vi "Main.vi"(11 "Module Admin":refnum<class "Delacor_lib_QMH_Cloneable Module Admin.lvclass">) -> ()   [LabVIEW 2024, in "Thermal Chamber.lvlib"]
doc: "This template is based off of the Queued Message Handler design pattern and the Queued Message Handler project template that ships with LabVIEW.\n\nThe main difference is that the queue is private to this module and communication between modules is performed via Broadcast and Request events.\n\nRequest events are wrapped in public API methods and are handled in the Event Handling Loop (EHL) of this VI. Any module can register for Broadcast events sent by this module. The EHL generates messages based on user interface actions.\n\nThe Message Handling Loop (MHL) processes messages generated by the EHL, or by other messages. The messages are string values, so new messages can be added easily to the Message Cases case structure in the MHL. Each message cluster can also provide an optional value for Message Data, which is a variant that can be converted to whatever message-specific data is required.\n_____\nBased on DQMH Project Template 6.0.0.91.\n\n<b>Note:</b> This VI was modified by the <b>Validate DQMH Module</b> tool to add a 'Panel Hidden' status updated broadcast to the Panel Close? event when External Launch = TRUE.\n\n<b>Note:</b> This VI was modified by the <b>Validate DQMH Module</b> tool to add a call to the Error Reported VI at the end of the 'Exit' MHL frame."
uses:
  Thermal Chamber.lvlib
  <vilib>/Delacor/Delacor QMH/Libraries/Cloneable Module Admin_class/Delacor_lib_QMH_Cloneable Module Admin.lvclass
  C:/Program Files/National Instruments/LabVIEW 2024/vi.lib/Delacor/Delacor QMH/Libraries/Module Admin_class/Delacor_lib_QMH_Module Admin.lvclass
  Module Data--cluster.ctl
  Class Libraries/Process Controller/_Thermal Process Controller.lvclass
  <vilib>/Delacor/Delacor QMH/Libraries/Message Queue_class/Delacor_lib_QMH_Message Queue.lvclass/Delacor_lib_QMH_Message Queue.ctl
  <vilib>/Delacor/Delacor QMH/Libraries/Cloneable Module Admin_class/Delacor_lib_QMH_Cloneable Module Admin.lvclass/Delacor_lib_QMH_Cloneable Module Admin.ctl
  Stop Argument--cluster.ctl
  <vilib>/Delacor/Delacor QMH/Libraries/Module Admin_class/Delacor_lib_QMH_Module Admin.lvclass/Delacor_lib_QMH_Module Admin.ctl
  Initialize Argument--cluster.ctl
  Class Libraries/Process Controller/Controls/Class Selector--Enum.ctl
  Initialize (Reply Payload)--cluster.ctl
  Shutdown Argument--cluster.ctl
  Shutdown (Reply Payload)--cluster.ctl
  Set Temp Setpoint Argument--cluster.ctl
  Class Libraries/Process Controller/Controls/Temp Data--Cluster.ctl
  Class Libraries/Process Controller/Controls/Temperature Units--Enum.ctl
  Set Temp Setpoint (Reply Payload)--cluster.ctl
  Set Temp Ramp Rate Argument--cluster.ctl
  Class Libraries/Process Controller/Controls/Temp Ramp Rate Data--Cluster.ctl
  Class Libraries/Process Controller/Controls/Rate Units--Enum.ctl
  Set Temp Ramp Rate (Reply Payload)--cluster.ctl
  Set Temp Control State Argument--cluster.ctl
  Set Temp Control State (Reply Payload)--cluster.ctl
  Get Temp Feedback Argument--cluster.ctl
  Get Temp Feedback (Reply Payload)--cluster.ctl
  Read Controller Data Argument--cluster.ctl
  Read Controller Data (Reply Payload)--cluster.ctl
  <vilib>/Utility/miscctls.llb/LVPointTypeDef.ctl
  Class Libraries/Simulated Process Controller/Simulated Thermal Process Controller.lvclass
  C:/Users/ghahn/OneDrive - Milwaukee Tool/Documents/LabVIEW Data/CML DQMH/Libraries/Thermal Chamber/Class Libraries/Process Controller/_Thermal Process Controller.lvclass
  Class Libraries/Watlow F4T/Watlow F4T.lvclass
  <vilib>/Delacor/Delacor QMH/Libraries/Message Queue_class/Delacor_lib_QMH_Enqueue Message (Single).vi
  <vilib>/Delacor/Delacor QMH/Libraries/Cloneable Module Admin_class/Delacor_lib_QMH_Get Module ID.vi
  <vilib>/Delacor/Delacor QMH/Libraries/Module Admin_class/Delacor_lib_QMH_Get External Launch.vi
  <vilib>/Utility/error.llb/Error Cluster From Error Code.vi
  <vilib>/ErrorRing/Error Ring.xnode
  <vilib>/Delacor/Delacor QMH/Libraries/Message Queue_class/Delacor_lib_QMH_Message Queue.lvclass
panel:
  out "Module ID":i32=-1
  out "error out":errorcluster
  out "Status":string
  in  "Simulate EHL Error":bool
  in  "Simulate MHL Error":bool
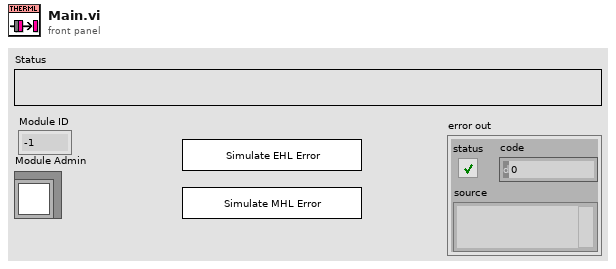
[diagram p1: front panel]
types:
  T1 = typedef "Thermal Chamber.lvlib/Request Events--cluster.ctl" = cluster{"Stop Module":refnum<user-event>, "Show Panel":refnum<user-event>, "Hide Panel":refnum<user-event>, "Show Diagram":refnum<user-event>, "Get Module Execution Status":refnum<user-event>, "Initialize":refnum<user-event>, "Shutdown":refnum<user-event>, "Set Temp Setpoint":refnum<user-event>, "Set Temp Ramp Rate":refnum<user-event>, "Set Temp Control State":refnum<user-event>, "Get Temp Feedback":refnum<user-event>, "Read Controller Data":refnum<user-event>}
  T2 = typedef "Thermal Chamber.lvlib/Module Data--cluster.ctl" = cluster{"Status":string, "_Thermal Process Controller":refnum<class "_Thermal Process Controller.lvclass">}
  T3 = enum32{"invalid lock state", "Not Locked", "Locked (No Password)", "Password-protected"}
  T4 = typedef "Thermal Chamber.lvlib/Stop Argument--cluster.ctl" = cluster{"Module ID":i32, "Origin":string, "Exit via Stop Module Req?":bool, "Wait for Module to stop?":bool}
  T5 = typedef "Thermal Chamber.lvlib/Initialize Argument--cluster.ctl" = cluster{"Module ID":i32, "Class Types":T6, "VISA":refnum<visa-resource-name>, "Wait Notifier":refnum<notifier>, "wait for reply":bool}
  T6 = typedef "_Thermal Process Controller.lvclass/Class Selector--Enum.ctl" = enum16{"Simulated Thermal Process Controller", "Watlow F4T"}
  T7 = typedef "Thermal Chamber.lvlib/Shutdown Argument--cluster.ctl" = cluster{"Module ID":i32, "Wait Notifier":refnum<notifier>, "wait for reply":bool}
  T8 = typedef "Thermal Chamber.lvlib/Set Temp Setpoint Argument--cluster.ctl" = cluster{"Module ID":i32, "Temp Setpoint Data":T9, "Wait Notifier":refnum<notifier>, "wait for reply":bool}
  T9 = typedef "_Thermal Process Controller.lvclass/Temp Data--Cluster.ctl" = cluster{"Temp":dbl, "Temp Units":T10}
  T10 = typedef "_Thermal Process Controller.lvclass/Temperature Units--Enum.ctl" = enum16{"Degrees F", "Degrees C", "Degrees K"}
  T11 = typedef "Thermal Chamber.lvlib/Set Temp Ramp Rate Argument--cluster.ctl" = cluster{"Module ID":i32, "Temp Ramp Data":T12, "Wait Notifier":refnum<notifier>, "wait for reply":bool}
  T12 = typedef "_Thermal Process Controller.lvclass/Temp Ramp Rate Data--Cluster.ctl" = cluster{"Temp Ramp Rate":dbl, "Temp Units":T10, "Rate Units":T13}
  T13 = typedef "_Thermal Process Controller.lvclass/Rate Units--Enum.ctl" = enum16{"Degrees/Minutes", "Degrees/Hours"}
  T14 = typedef "Thermal Chamber.lvlib/Set Temp Control State Argument--cluster.ctl" = cluster{"Module ID":i32, "State":bool, "Wait Notifier":refnum<notifier>, "wait for reply":bool}
  T15 = typedef "Thermal Chamber.lvlib/Get Temp Feedback Argument--cluster.ctl" = cluster{"Module ID":i32, "Temp Units":T10, "Wait Notifier":refnum<notifier>, "wait for reply":bool}
  T16 = typedef "Thermal Chamber.lvlib/Read Controller Data Argument--cluster.ctl" = cluster{"Module ID":i32, "Temp Units":T10, "Wait Notifier":refnum<notifier>, "wait for reply":bool}
  T17 = typedef "LVPointTypeDef.ctl" = cluster{"Horizontal":i16, "Vertical":i16}
  T18 = enum32{"Invalid", "Standard", "Closed", "Hidden", "Minimized", "Maximized"}
  T19 = typedef "Thermal Chamber.lvlib/Initialize (Reply Payload)--cluster.ctl" = cluster{"Module ID":i32, "Ready":bool, "error":errorcluster}
  T20 = typedef "Thermal Chamber.lvlib/Shutdown (Reply Payload)--cluster.ctl" = cluster{"Module ID":i32, "Shutdown?":bool, "error":errorcluster}
  T21 = typedef "Thermal Chamber.lvlib/Set Temp Setpoint (Reply Payload)--cluster.ctl" = cluster{"Set?":bool, "Temp Setpoint Data":T9, "error":errorcluster, "Module ID":i32}
  T22 = typedef "Thermal Chamber.lvlib/Set Temp Ramp Rate (Reply Payload)--cluster.ctl" = cluster{"Set?":bool, "Temp Ramp Data":T12, "error":errorcluster, "Module ID":i32}
  T23 = typedef "Thermal Chamber.lvlib/Set Temp Control State (Reply Payload)--cluster.ctl" = cluster{"Set?":bool, "State":bool, "error":errorcluster, "Module ID":i32}
  T24 = typedef "Thermal Chamber.lvlib/Get Temp Feedback (Reply Payload)--cluster.ctl" = cluster{"Temp Feedback Data":T9, "error":errorcluster, "Module ID":i32}
  T25 = typedef "Thermal Chamber.lvlib/Read Controller Data (Reply Payload)--cluster.ctl" = cluster{"Chamber Temp":T9, "Temp Setpoint":T9, "Chamber Output":dbl, "error":errorcluster, "Module ID":i32}
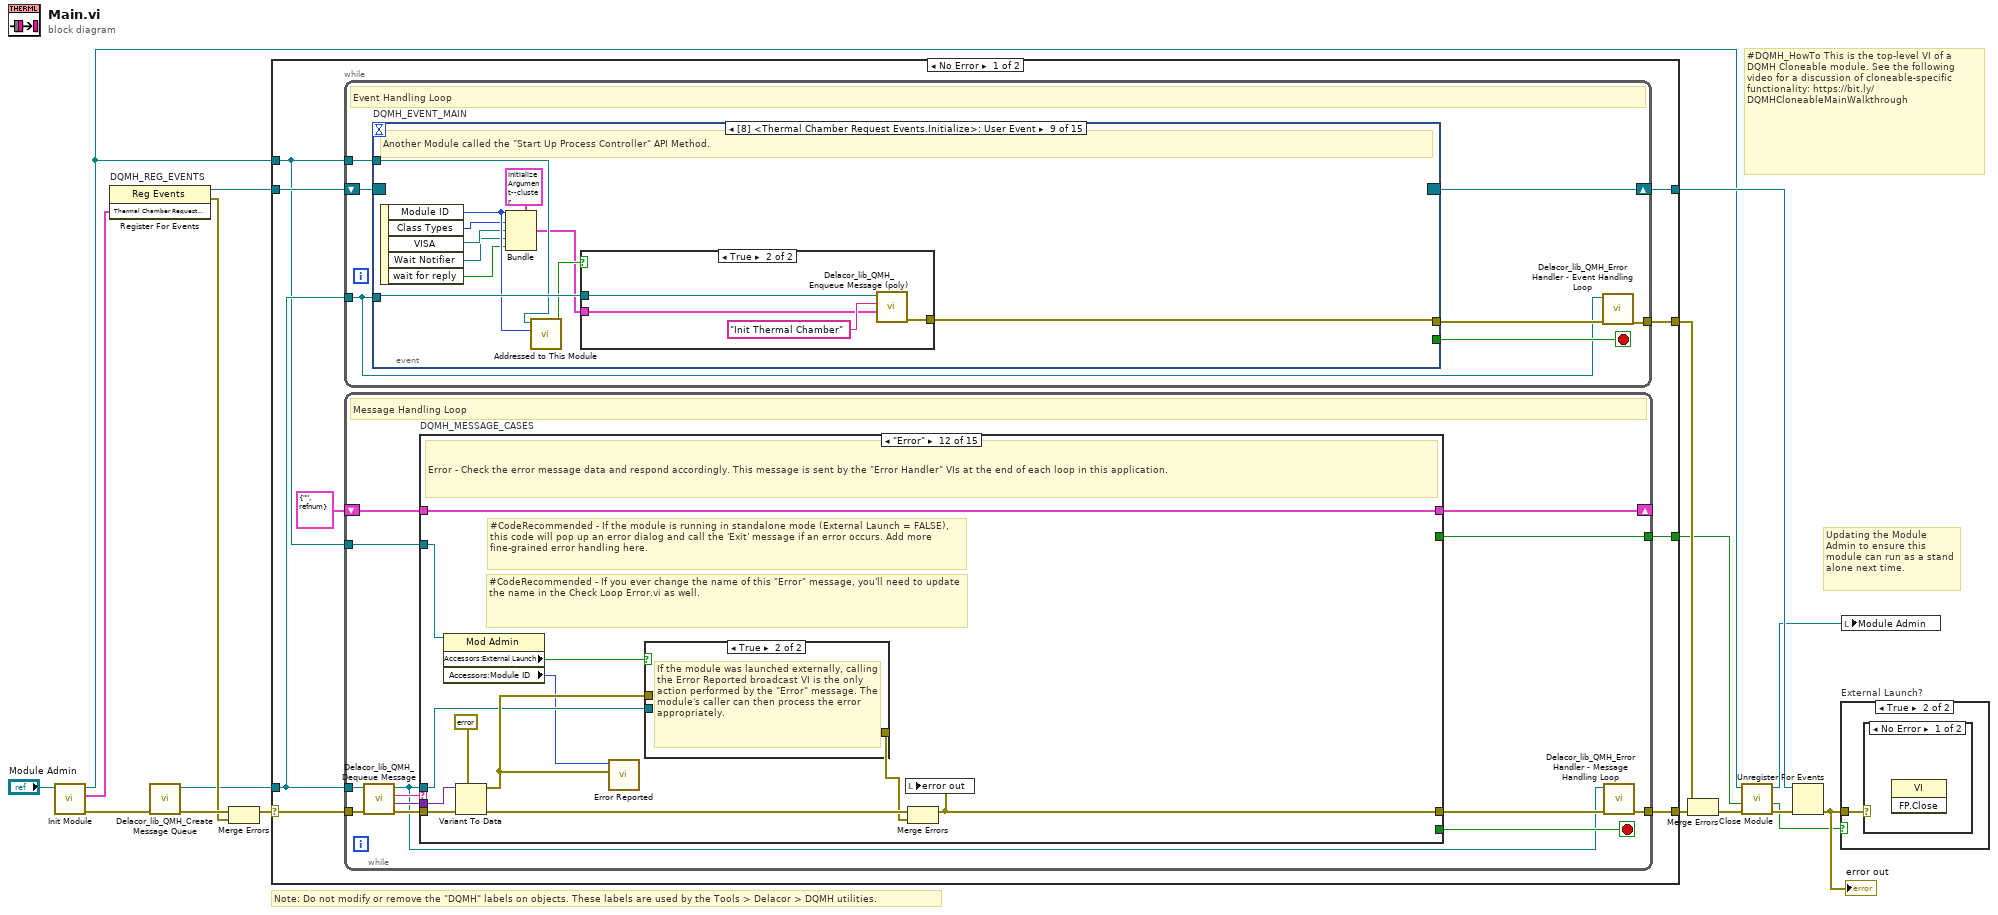
[diagram p0: block diagram]
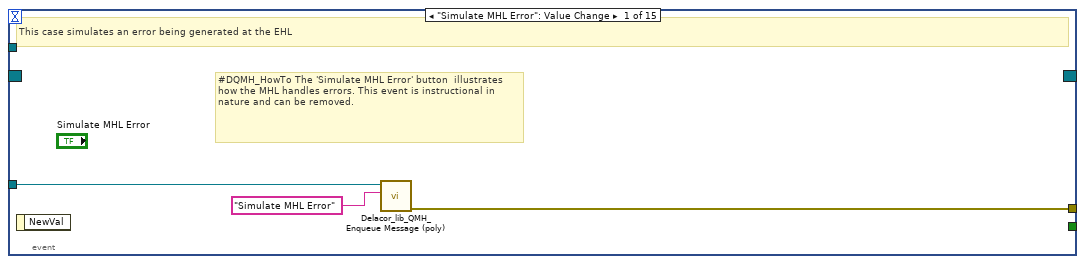
[diagram p2: hidden frame]
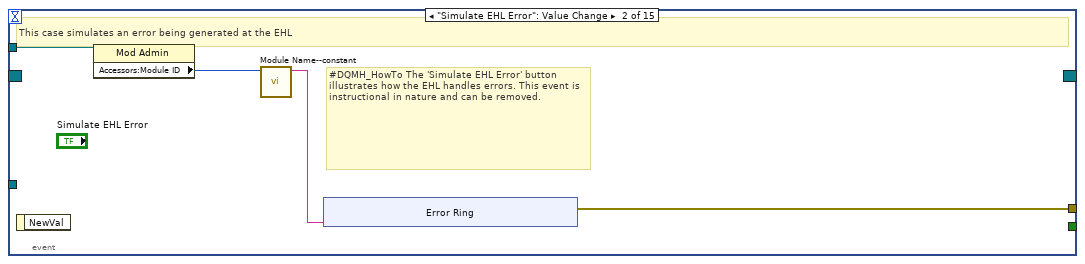
[diagram p3: hidden frame]
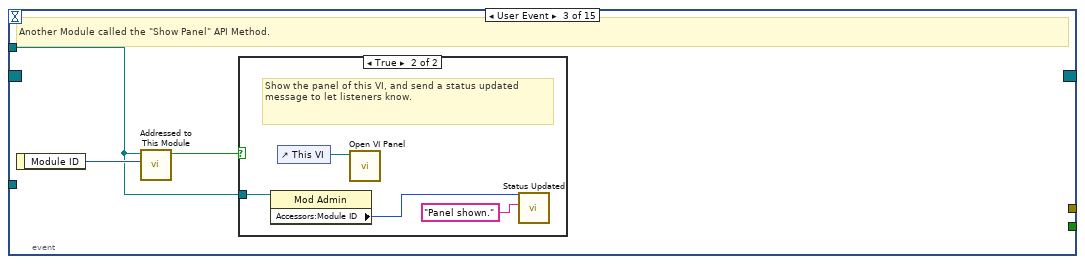
[diagram p4: hidden frame]
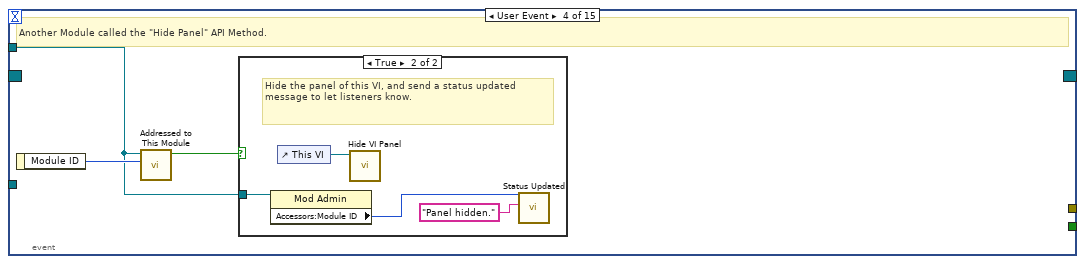
[diagram p6: hidden frame]
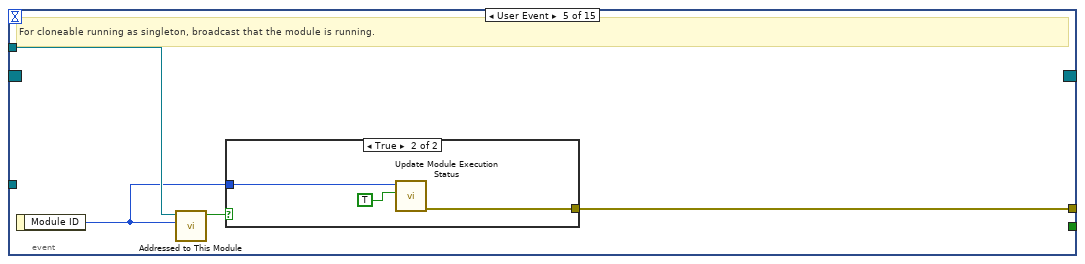
[diagram p8: hidden frame]
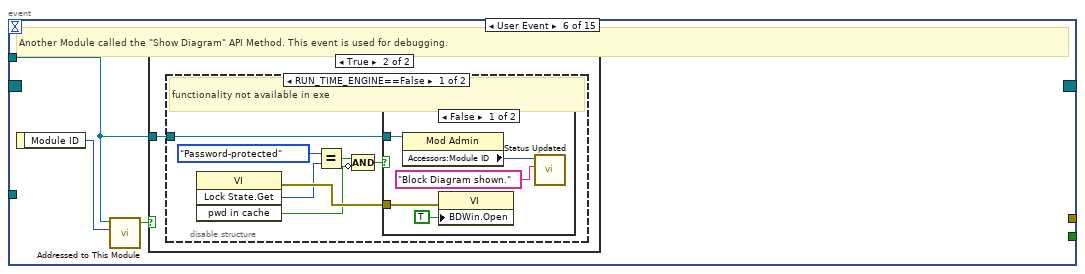
[diagram p10: hidden frame]
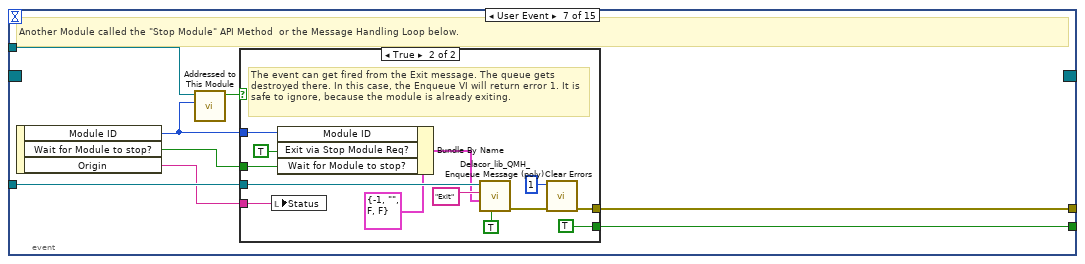
[diagram p14: hidden frame]
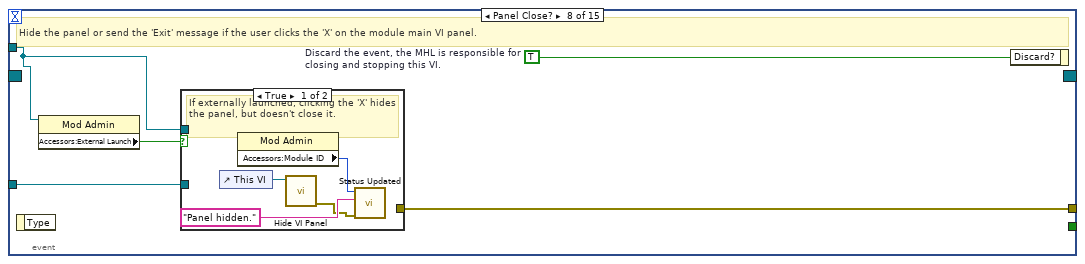
[diagram p16: hidden frame]
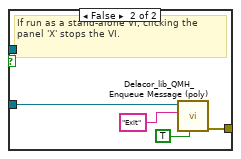
[diagram p17: hidden frame]
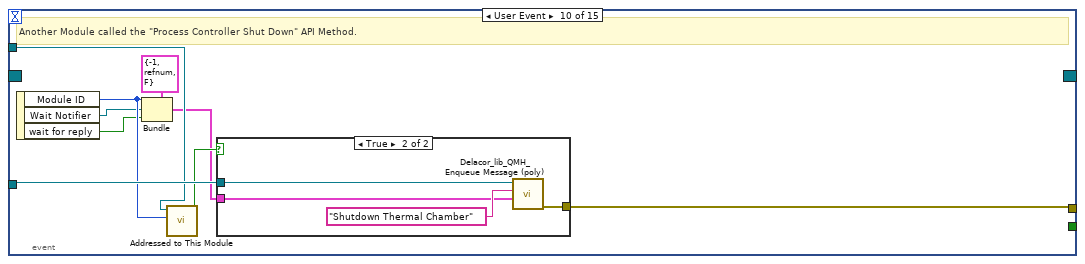
[diagram p19: hidden frame]
diagram:
  # "#DQMH_HowTo This is the top-level VI of a DQMH Cloneable module. See the following video for a discussion of cloneable-specific functionality: https://bit.ly/DQMHCloneableMainWalkthrough"
  # "Note: Do not modify or remove the \"DQMH\" labels on objects. These labels are used by the Tools > Delacor > DQMH utilities."
  # "Updating the Module Admin to ensure this module can run as a stand alone next time."
  n1 = call "Init Module.vi"("Cloneable Module Admin in"="Module Admin") -> ("error out"=w15:errorcluster, "Thermal Chamber Request Events"=w7:T1, "Cloneable Module Admin out"=w4:refnum<class "Delacor_lib_QMH_Cloneable Module Admin.lvclass">)  [unwired: 8 in]
  n2 = register-events "DQMH_REG_EVENTS"(w7) -> (reference out=w8:refnum<event-registration>, error out=w10:errorcluster)  [unwired: 2 in]
  n3 = call <vilib>:"Delacor_lib_QMH_Create Message Queue.vi"("error in"=w15) -> ("error out"=w12:errorcluster, "Message Queue"=w6:refnum<class "Delacor_lib_QMH_Message Queue.lvclass">)  [unwired: 9 in]
  n4 = Merge Errors(w12, w10) -> (w11:errorcluster)
  n5 = case shown="No Error" w11 {
    selector: w11 -> [w25 w508]
    tunnel: [w27 w507] -> w16
    tunnel: [w24 w515] -> w9
    tunnel: w8 -> [w22 w515]
    tunnel: w6 -> [w21 w506]
    tunnel: [w26 _] -> w17
    tunnel: w4 -> [w20 w511]
    tunnel: [w19 _] -> w2
    frame No Error {
      n6 = while {
        tunnel: w21 -> [w28]
        shift-right: [w31] -> w24
        shift-left: w22 -> [w32]
        tunnel: [w33] -> w26
        tunnel: w20 -> [w29]
        stop <- w30 stop-if-true
        # "Event Handling Loop"
        n7 = event "DQMH_EVENT_MAIN" shown="[8] <Thermal Chamber Request Events.Initialize>: User Event" {
          selector: w32 -> [_ _ _ _ _ _ _ _ _ _ _ _ _ _ _]
          dyn-events: [_ _ _ _ _ _ _ _ _ _ _ _ _ _ _] -> w31
          timeout: _ -> [_ _ _ _ _ _ _ _ _ _ _ _ _ _ _]
          tunnel: [_ _ _ _ _ _ w89 _ _ _ _ _ _ _ _] -> w30
          tunnel: w28 -> [w36 _ _ _ _ _ w92 w109 w131 w144 w158 w172 w186 w200 w214]
          tunnel: [w37 w41 _ _ w66 _ w93 w111 w124 w136 w149 w163 w177 w191 w207] -> w34
          tunnel: w29 -> [_ w40 w49 w56 w64 w70 w91 w107 w129 w142 w156 w170 w184 w198 w212]
          event "Simulate MHL Error": Value Change {
            # "#DQMH_HowTo The 'Simulate MHL Error' button  illustrates how the MHL handles errors. This event is instructional in nature and can be removed."
            # "This case simulates an error being generated at the EHL"
            n8 = event-data() -> ()  [unwired: 1 in, 1 out]
            n9 = call-poly <vilib>:"Delacor_lib_QMH_Enqueue Message (poly).vi"("Message"="Simulate MHL Error", "Message Queue in"=w36) -> ("error out"=w37:errorcluster)  [unwired: 8 in, 1 out]
          }
          event "Simulate EHL Error": Value Change {
            # "#DQMH_HowTo The 'Simulate EHL Error' button  illustrates how the EHL handles errors. This event is instructional in nature and can be removed."
            # "This case simulates an error being generated at the EHL"
            n10 = event-data() -> ()  [unwired: 1 in, 1 out]
            n11 = property on="Property Node" class="Mod Admin"(reference=w40) -> ("Accessors:Module ID"=w39:i32)  [unwired: 1 in, 2 out]
            n12 = call "Module Name--constant.vi"("Module ID"=w39) -> ("Module Name"=w38:string)  [unwired: 10 in]
            n13 = xnode "Error Ring"("parameter 0"=w38) -> ("error out"=w41:errorcluster)
          }
          event User Event {
            # "Another Module called the \"Show Panel\" API Method."
            n14 = event-data() -> ("Module ID"=w50:i32)  [unwired: 1 in]
            n15 = call "Addressed to This Module.vi"("Module ID from Argument"=w50, "Module Admin"=w49) -> ("Addressed to this instance?"=w51:bool)  [unwired: 8 in, 1 out]
            n16 = case shown="True" w51 {
              tunnel: w49 -> [_ w53]
              frame False {
              }
              frame True {
                # "Show the panel of this VI, and send a status updated message to let listeners know."
                n17 = property on="Property Node" class="Mod Admin"(reference=w53) -> ("Accessors:Module ID"=w52:i32)  [unwired: 1 in, 2 out]
                n18 = control-ref of="This VI"() -> (w55:refnum<vi>)
                n19 = call "Open VI Panel.vi"("VI"=w55) -> ()  [unwired: 10 in, 1 out]
                n20 = call "Status Updated.vi"("Status"="Panel shown." ("format string"), "Module ID"=w52) -> ()  [unwired: 9 in, 1 out]
              }
            }
          }
          event User Event {
            # "Another Module called the \"Hide Panel\" API Method."
            n21 = event-data() -> ("Module ID"=w57:i32)  [unwired: 1 in]
            n22 = call "Addressed to This Module.vi"("Module ID from Argument"=w57, "Module Admin"=w56) -> ("Addressed to this instance?"=w58:bool)  [unwired: 8 in, 1 out]
            n23 = case shown="True" w58 {
              tunnel: w56 -> [_ w60]
              frame False {
              }
              frame True {
                # "Hide the panel of this VI, and send a status updated message to let listeners know."
                n24 = property on="Property Node" class="Mod Admin"(reference=w60) -> ("Accessors:Module ID"=w59:i32)  [unwired: 1 in, 2 out]
                n25 = control-ref of="This VI"() -> (w62:refnum<vi>)
                n26 = call "Hide VI Panel.vi"("VI"=w62) -> ()  [unwired: 10 in, 1 out]
                n27 = call "Status Updated.vi"("Status"="Panel hidden." ("format string"), "Module ID"=w59) -> ()  [unwired: 9 in, 1 out]
              }
            }
          }
          event User Event {
            # "For cloneable running as singleton, broadcast that the module is running."
            n28 = event-data() -> ("Module ID"=w63:i32)  [unwired: 1 in]
            n29 = call "Addressed to This Module.vi"("Module ID from Argument"=w63, "Module Admin"=w64) -> ("Addressed to this instance?"=w65:bool)  [unwired: 8 in, 1 out]
            n30 = case shown="True" w65 {
              tunnel: [_ w69] -> w66
              tunnel: w63 -> [_ w68]
              frame False {
              }
              frame True {
                n31 = call "Update Module Execution Status.vi"("Running?"=TRUE, "Module ID"=w68) -> ("error out"=w69:errorcluster)  [unwired: 9 in]
              }
            }
          }
          event User Event {
            # "Another Module called the \"Show Diagram\" API Method. This event is used for debugging."
            n32 = event-data() -> ("Module ID"=w71:i32)  [unwired: 1 in]
            n33 = call "Addressed to This Module.vi"("Module ID from Argument"=w71, "Module Admin"=w70) -> ("Addressed to this instance?"=w72:bool)  [unwired: 8 in, 1 out]
            n34 = case shown="True" w72 {
              tunnel: w70 -> [_ w73]
              frame False {
              }
              frame True {
                n35 = disable-structure shown="RUN_TIME_ENGINE==False" {
                  disable-tunnel: w73 -> [w74 _]
                  frame condition #0 (active) {
                    # "functionality not available in exe"
                    n36 = invoke on="Invoke Node" class="VI" method="Lock State.Get"() -> (error out=w80:errorcluster, "Get Lock State"=w79:T3, "pwd in cache"=w76:bool)  [unwired: 4 in, 1 out]
                    n37 = Equal?(x=T3."Password-protected", y=w79) -> (x = y?=w77:bool)
                    n38 = Compound Arithmetic op=AND(w77, invert w76) -> (w75:bool)
                    n39 = case shown="False" w75 {
                      tunnel: w80 -> [w85 _]
                      tunnel: w74 -> [w82 _]
                      frame False {
                        n40 = property on="Property Node" class="Mod Admin"(reference=w82) -> ("Accessors:Module ID"=w81:i32)  [unwired: 1 in, 2 out]
                        n41 = property on="Property Node" class="VI"(error in=w85, "BDWin.Open"=TRUE ("Block Diagram Window:Open")) -> ()  [unwired: 1 in, 2 out]
                        n42 = call "Status Updated.vi"("Status"="Block Diagram shown." ("format string"), "Module ID"=w81) -> ()  [unwired: 9 in, 1 out]
                      }
                      frame True {
                        # "Password-protected VI, and the password is not in the cache. Do not show the diagram."
                      }
                    }
                  }
                  frame condition #1 {
                  }
                }
              }
            }
          }
          event User Event {
            # "Another Module called the \"Stop Module\" API Method  or the Message Handling Loop below."
            n43 = event-data() -> ("Module ID"=w87:i32, "Wait for Module to stop?"=w88:bool, "Origin"=w86:string)  [unwired: 1 in]
            n44 = call "Addressed to This Module.vi"("Module ID from Argument"=w87, "Module Admin"=w91) -> ("Addressed to this instance?"=w90:bool)  [unwired: 8 in, 1 out]
            n45 = case shown="True" w90 {
              tunnel: [_ w105] -> w93
              tunnel: w92 -> [_ w101]
              tunnel: [_ TRUE] -> w89
              tunnel: w88 -> [_ w96]
              tunnel: w87 -> [_ w98]
              tunnel: w86 -> [_ w94]
              frame False {
              }
              frame True {
                # "The event can get fired from the Exit message. The queue gets destroyed there. In this case, the Enqueue VI will return error 1. It is safe to ignore, because the module is already exiting."
                n46 = local write "Status"(w94) -> ()
                n47 = Bundle By Name(cluster=T4 {"Module ID"=-1, "Origin"="", "Exit via Stop Module Req?"=FALSE, "Wait for Module to stop?"=FALSE} ("Stop Argument"), "Module ID"=w98, "Exit via Stop Module Req?"=TRUE, "Wait for Module to stop?"=w96) -> (w95:T4)
                n48 = call-poly <vilib>:"Delacor_lib_QMH_Enqueue Message (poly).vi"("Priority Message? (F)"=TRUE, "Message Data"=w95, "Message"="Exit", "Message Queue in"=w101) -> ("error out"=w106:errorcluster)  [unwired: 6 in, 1 out]
                n49 = call <vilib>:"Clear Errors.vi"("error in (no error)"=w106, "specific error code to clear (0: all)"=1) -> ("error out"=w105:errorcluster)  [unwired: 4 in, 1 out]
              }
            }
          }
          event Panel Close? {
            w110 = TRUE  # Discard the event, the MHL is responsible for closing and stopping this VI.
            # "Hide the panel or send the 'Exit' message if the user clicks the 'X' on the module main VI panel."
            n50 = event-data() -> ()  [unwired: 1 in, 1 out]
            n51 = property on="Property Node" class="Mod Admin"(reference=w107) -> ("Accessors:External Launch"=w108:bool)  [unwired: 1 in, 2 out]
            n52 = case shown="True" w108 {
              tunnel: w109 -> [_ w119]
              tunnel: [_ w120] -> w111
              tunnel: w107 -> [w114 _]
              frame True {
                # "If externally launched, clicking the 'X' hides the panel, but doesn't close it."
                n53 = control-ref of="This VI"() -> (w116:refnum<vi>)
                n54 = property class="Mod Admin"(reference=w114) -> ("Accessors:Module ID"=w113:i32)  [unwired: 1 in, 2 out]
                n55 = call "Hide VI Panel.vi"("VI"=w116) -> ("error out"=w112:errorcluster)  [unwired: 10 in]
                n56 = call "Status Updated.vi"("error in (no error)"=w112, "Status"="Panel hidden.", "Module ID"=w113) -> ()  [unwired: 8 in, 1 out]
              }
              frame False {
                # "If run as a stand-alone VI, clicking the panel 'X' stops the VI."
                n57 = call-poly <vilib>:"Delacor_lib_QMH_Enqueue Message (poly).vi"("Priority Message? (F)"=TRUE, "Message"="Exit", "Message Queue in"=w119) -> ("error out"=w120:errorcluster)  [unwired: 7 in, 1 out]
              }
            }
            n58 = event-data ("Event Filter Node")("Discard?"=w110) -> ()  [unwired: 1 in, 1 out]
          }
          event User Event {
            # "Another Module called the \"Start Up Process Controller\" API Method."
            n59 = event-data() -> ("Module ID"=w126:i32, "Class Types"=w125:T6, "VISA"=w123:refnum<visa-resource-name>, "Wait Notifier"=w122:refnum<notifier>, "wait for reply"=w121:bool)  [unwired: 1 in]
            n60 = Bundle(cluster=T5 {"Module ID"=-1, "Class Types"=enum."Simulated Thermal Process Controller", "VISA"="", "Wait Notifier"=refnum, "wait for reply"=FALSE} ("Start Up Process Controller Argument"), "Module ID"=w126, "Class Types"=w125, "VISA"=w123, "Wait Notifier"=w122, "wait for reply"=w121) -> (w127:T5)
            n61 = call "Addressed to This Module.vi"("Module ID from Argument"=w126, "Module Admin"=w129) -> ("Addressed to this instance?"=w130:bool)  [unwired: 8 in, 1 out]
            n62 = case shown="True" w130 {
              tunnel: w131 -> [_ w135]
              tunnel: w127 -> [_ w133]
              tunnel: [_ w132] -> w124
              frame False {
              }
              frame True {
                n63 = call-poly <vilib>:"Delacor_lib_QMH_Enqueue Message (poly).vi"("Message Data"=w133, "Message"="Init Thermal Chamber", "Message Queue in"=w135) -> ("error out"=w132:errorcluster)  [unwired: 7 in, 1 out]
              }
            }
          }
          event User Event {
            # "Another Module called the \"Process Controller Shut Down\" API Method."
            n64 = event-data() -> ("Module ID"=w139:i32, "Wait Notifier"=w138:refnum<notifier>, "wait for reply"=w137:bool)  [unwired: 1 in]
            n65 = Bundle(cluster=T7 {"Module ID"=-1, "Wait Notifier"=refnum, "wait for reply"=FALSE} ("Process Controller Shut Down Argument"), "Module ID"=w139, "Wait Notifier"=w138, "wait for reply"=w137) -> (w140:T7)
            n66 = call "Addressed to This Module.vi"("Module ID from Argument"=w139, "Module Admin"=w142) -> ("Addressed to this instance?"=w143:bool)  [unwired: 8 in, 1 out]
            n67 = case shown="True" w143 {
              tunnel: w144 -> [_ w148]
              tunnel: w140 -> [_ w146]
              tunnel: [_ w145] -> w136
              frame False {
              }
              frame True {
                n68 = call-poly <vilib>:"Delacor_lib_QMH_Enqueue Message (poly).vi"("Message Data"=w146, "Message"="Shutdown Thermal Chamber", "Message Queue in"=w148) -> ("error out"=w145:errorcluster)  [unwired: 7 in, 1 out]
              }
            }
          }
          event User Event {
            # "Another Module called the \"Set Temp Setpoint\" API Method."
            n69 = event-data() -> ("Module ID"=w153:i32, "Temp Setpoint Data"=w152:T9, "Wait Notifier"=w151:refnum<notifier>, "wait for reply"=w150:bool)  [unwired: 1 in]
            n70 = Bundle(cluster=T8 {"Module ID"=-1, "Temp Setpoint Data"={"Temp"=0.0, "Temp Units"=enum."Degrees F"}, "Wait Notifier"=refnum, "wait for reply"=FALSE} ("Set Temp Setpoint Argument"), "Module ID"=w153, "Temp Setpoint Data"=w152, "Wait Notifier"=w151, "wait for reply"=w150) -> (w154:T8)
            n71 = call "Addressed to This Module.vi"("Module ID from Argument"=w153, "Module Admin"=w156) -> ("Addressed to this instance?"=w157:bool)  [unwired: 8 in, 1 out]
            n72 = case shown="True" w157 {
              tunnel: w158 -> [_ w162]
              tunnel: w154 -> [_ w160]
              tunnel: [_ w159] -> w149
              frame False {
              }
              frame True {
                n73 = call-poly <vilib>:"Delacor_lib_QMH_Enqueue Message (poly).vi"("Message Data"=w160, "Message"="Set Temp Setpoint", "Message Queue in"=w162) -> ("error out"=w159:errorcluster)  [unwired: 7 in, 1 out]
              }
            }
          }
          event User Event {
            # "Another Module called the \"Set Temp Ramp Rate\" API Method."
            n74 = event-data() -> ("Module ID"=w167:i32, "Temp Ramp Data"=w166:T12, "Wait Notifier"=w165:refnum<notifier>, "wait for reply"=w164:bool)  [unwired: 1 in]
            n75 = Bundle(cluster=T11 {"Module ID"=-1, "Temp Ramp Data"={"Temp Ramp Rate"=0.0, "Temp Units"=enum."Degrees F", "Rate Units"=enum."Degrees/Minutes"}, "Wait Notifier"=refnum, "wait for reply"=FALSE} ("Set Temp Ramp Rate Argument"), "Module ID"=w167, "Temp Ramp Data"=w166, "Wait Notifier"=w165, "wait for reply"=w164) -> (w168:T11)
            n76 = call "Addressed to This Module.vi"("Module ID from Argument"=w167, "Module Admin"=w170) -> ("Addressed to this instance?"=w171:bool)  [unwired: 8 in, 1 out]
            n77 = case shown="True" w171 {
              tunnel: w172 -> [_ w176]
              tunnel: w168 -> [_ w174]
              tunnel: [_ w173] -> w163
              frame False {
              }
              frame True {
                n78 = call-poly <vilib>:"Delacor_lib_QMH_Enqueue Message (poly).vi"("Message Data"=w174, "Message"="Set Temp Ramp Rate", "Message Queue in"=w176) -> ("error out"=w173:errorcluster)  [unwired: 7 in, 1 out]
              }
            }
          }
          event User Event {
            # "Another Module called the \"Set Temp Control State\" API Method."
            n79 = event-data() -> ("Module ID"=w181:i32, "State"=w180:bool, "Wait Notifier"=w179:refnum<notifier>, "wait for reply"=w178:bool)  [unwired: 1 in]
            n80 = Bundle(cluster=T14 {"Module ID"=-1, "State"=FALSE, "Wait Notifier"=refnum, "wait for reply"=FALSE} ("Set Temp Control State Argument"), "Module ID"=w181, "State"=w180, "Wait Notifier"=w179, "wait for reply"=w178) -> (w182:T14)
            n81 = call "Addressed to This Module.vi"("Module ID from Argument"=w181, "Module Admin"=w184) -> ("Addressed to this instance?"=w185:bool)  [unwired: 8 in, 1 out]
            n82 = case shown="True" w185 {
              tunnel: w186 -> [_ w190]
              tunnel: w182 -> [_ w188]
              tunnel: [_ w187] -> w177
              frame False {
              }
              frame True {
                n83 = call-poly <vilib>:"Delacor_lib_QMH_Enqueue Message (poly).vi"("Message Data"=w188, "Message"="Set Temp Control State", "Message Queue in"=w190) -> ("error out"=w187:errorcluster)  [unwired: 7 in, 1 out]
              }
            }
          }
          event User Event {
            # "Another Module called the \"Get Temp Feedback\" API Method."
            n84 = event-data() -> ("Module ID"=w195:i32, "Temp Units"=w194:T10, "Wait Notifier"=w193:refnum<notifier>, "wait for reply"=w192:bool)  [unwired: 1 in]
            n85 = Bundle(cluster=T15 {"Module ID"=-1, "Temp Units"=enum."Degrees F", "Wait Notifier"=refnum, "wait for reply"=FALSE} ("Get Temp Feedback Argument"), "Module ID"=w195, "Temp Units"=w194, "Wait Notifier"=w193, "wait for reply"=w192) -> (w196:T15)
            n86 = call "Addressed to This Module.vi"("Module ID from Argument"=w195, "Module Admin"=w198) -> ("Addressed to this instance?"=w199:bool)  [unwired: 8 in, 1 out]
            n87 = case shown="True" w199 {
              tunnel: w200 -> [_ w204]
              tunnel: w196 -> [_ w202]
              tunnel: [_ w201] -> w191
              frame False {
              }
              frame True {
                n88 = call-poly <vilib>:"Delacor_lib_QMH_Enqueue Message (poly).vi"("Message Data"=w202, "Message"="Get Temp Feedback", "Message Queue in"=w204) -> ("error out"=w201:errorcluster)  [unwired: 7 in, 1 out]
              }
            }
          }
          event User Event {
            # "Another Module called the \"Read Controller Data\" API Method."
            n89 = event-data() -> ("Module ID"=w209:i32, "Temp Units"=w208:T10, "Wait Notifier"=w205:refnum<notifier>, "wait for reply"=w206:bool)  [unwired: 1 in]
            n90 = Bundle(cluster=T16 {"Module ID"=-1, "Temp Units"=enum."Degrees F", "Wait Notifier"=refnum, "wait for reply"=FALSE} ("Read Controller Data Argument"), "Module ID"=w209, "Temp Units"=w208, "Wait Notifier"=w205, "wait for reply"=w206) -> (w210:T16)
            n91 = call "Addressed to This Module.vi"("Module ID from Argument"=w209, "Module Admin"=w212) -> ("Addressed to this instance?"=w213:bool)  [unwired: 8 in, 1 out]
            n92 = case shown="True" w213 {
              tunnel: w214 -> [_ w218]
              tunnel: w210 -> [_ w216]
              tunnel: [_ w215] -> w207
              frame False {
              }
              frame True {
                n93 = call-poly <vilib>:"Delacor_lib_QMH_Enqueue Message (poly).vi"("Message Data"=w216, "Message"="Read Controller Data", "Message Queue in"=w218) -> ("error out"=w215:errorcluster)  [unwired: 7 in, 1 out]
              }
            }
          }
        }
        n94 = call-dynamic "Delacor_lib_QMH_Error Handler - Event Handling Loop.vi"("error in"=w34, "Message Queue in"=w28) -> ("dup error in"=w33:errorcluster)  [unwired: 8 in, 1 out]
      }
      n95 = while {
        tunnel: w21 -> [w222]
        shift-right: [w226] -> _
        shift-left: T2 {"Status"="", "_Thermal Process Controller"=refnum} ("Data Cluster") -> [w227]
        tunnel: w25 -> [w230]
        tunnel: [w228] -> w27
        tunnel: w20 -> [w220]
        tunnel: [w219] -> w19
        stop <- w225 stop-if-true
        # "Message Handling Loop"
        n96 = call-dynamic "Delacor_lib_QMH_Dequeue Message.vi"("error in"=w230, "Message Queue in"=w222) -> ("error out"=w229:errorcluster, "Message Data"=w223:variant, "Message"=w224:string, "Message Queue out"=w221:refnum<class "Delacor_lib_QMH_Message Queue.lvclass">)  [unwired: 6 in]
        n97 = case "DQMH_MESSAGE_CASES" shown="\"Error\"" w224 {
          selector: w224 -> [_ _ _ _ _ _ _ _ _ _ _ _ _ _ w493]
          tunnel: w221 -> [_ _ _ _ _ _ _ _ _ _ _ w443 _ w483 _]
          tunnel: w229 -> [w250 w254 w285 w309 w334 w358 w381 w403 w434 w439 w441 w452 w465 w489 w495]
          tunnel: [w248 w254 w272 w295 w315 w339 w364 w387 w408 w438 w441 w448 w464 w486 w496] -> w231
          tunnel: w227 -> [w241 w253 w269 w297 w324 w349 w369 w394 w425 w437 w440 w447 w462 w482 w494]
          tunnel: [w240 w253 w270 w298 w325 w350 w370 w393 w426 w437 w440 w447 w462 w482 w494] -> w226
          tunnel: [_ _ _ _ _ _ _ _ _ _ _ _ _ w481 _] -> w225
          tunnel: w223 -> [_ _ w284 w308 w333 w357 w380 w402 w433 _ _ w446 _ w479 _]
          tunnel: w220 -> [w235 _ _ _ w313 w337 w361 w384 w406 _ _ w445 w460 w475 w491]
          tunnel: [_ _ _ _ _ _ _ _ _ _ _ _ _ w477 _] -> w219
          frame "Initialize" {
            w232 = "Initial Message" ("Initial Message")
            # "#CodeNeeded - Initialize the appearance of the front panel."
            # "#CodeNeeded - Initialize your state data here."
            # "Initialize - Any operation that needs to be done before the module can receive messages. Synchronize Caller Events.vi will inform Start Module.vi that the module has launched and is ready to receive messages. Module Did Init.vi will broadcast that the module initialized."
            n98 = call "Synchronize Caller Events.vi"("error in (no error)"=w250, "Module Admin"=w235) -> ("error out"=w249:errorcluster, "Module Admin out"=w234:refnum<class "Delacor_lib_QMH_Cloneable Module Admin.lvclass">)  [unwired: 8 in]
            n99 = property on="Property Node" class="Mod Admin"(reference=w234) -> ("Accessors:Module ID"=w237:i32, "Accessors:External Launch"=w236:bool)  [unwired: 1 in, 2 out]
            "Module ID" <- w237
            n100 = call "Module Name--constant.vi"("Module ID"=w237) -> ("Module Name"=w245:string)  [unwired: 10 in]
            n101 = property on="Property Node" class="VI"("Front Panel.Title"=w245) -> (reference out=w247:refnum<vi>, error out=w252:errorcluster)  [unwired: 2 in]
            n102 = Select(t=T18."Hidden" ("State"), s=w236, f=T18."Standard" ("State")) -> (s? t:f=w242:T18)
            n103 = invoke on="Invoke Node" class="VI" method="FP.Open"(reference=w247, error in=w252, "State"=w242) -> (reference out=w246:refnum<vi>, error out=w251:errorcluster)  [unwired: 2 in, 3 out]
            n104 = call "Module Name--constant.vi"("Module ID"=w237) -> ("Module Name"=w238:string)  [unwired: 10 in]
            n105 = Bundle By Name(cluster=w241, "Status"=w232) -> (w240:T2)
            n106 = invoke on="Invoke Node" class="VI" method="FP.Center"(reference=w246, error in=w251) -> ()  [unwired: 1 in, 3 out]
            n107 = property on="Pane" class="Pane"("Origin"=T17 {"Horizontal"=0, "Vertical"=0}) -> ()  [unwired: 2 in, 2 out]
            n108 = call "Module Did Init.vi"("error in (no error)"=w249, "Initialized?"=TRUE, "Origin"=w238, "Module ID"=w237) -> ("error out"=w248:errorcluster)  [unwired: 7 in]
            "Status" <- w232
          }
          frame "---Module Specific---" {
            # "Separator -- The following cases handle messages specific to this Module."
          }
          frame "Init Thermal Chamber" {
            # "Perform start up operations (establish connection, load standby configurations) on the process controller"
            n109 = Variant To Data(error in=w285, type=T5 {"Module ID"=-1, "Class Types"=enum."Simulated Thermal Process Controller", "VISA"="", "Wait Notifier"=refnum, "wait for reply"=FALSE} ("Start Up Process Controller Argument"), Variant=w284) -> (data=w282:T5, error out=w275:errorcluster)
            n110 = Unbundle By Name(w282) -> ("Class Types"=w260:T6, "VISA"=w271:refnum<visa-resource-name>, "Wait Notifier"=w281:refnum<notifier>, "wait for reply"=w280:bool)
            n111 = Build Array(refnum<class "Watlow F4T.lvclass"> refnum ("Watlow F4T.lvclass"), refnum<class "Simulated Thermal Process Controller.lvclass"> refnum ("Simulated Thermal Process Controller.lvclass")) -> (w261:refnum<class "_Thermal Process Controller.lvclass">[])
            n112 = Format Into String(w260) -> (resulting string=w258:string)  [unwired: 3 in, 1 out]
            n113 = call "List Child Class Paths.vi"("[Class Objects]"=w261) -> ("Child Class Names"=w257:string[], "Child Class Paths"=w256:path[])  [unwired: 8 in, 1 out]
            n114 = for {
              tunnel: w257 -> [w290] mode=indexing
              tunnel: w258 -> [w289]
              tunnel: [w286] -> w259
              i -> [w286]
              stop <- w287 stop-if-true
              n115 = Match Pattern(string=w290, regular expression=w289) -> (offset past match=w288:i32)  [unwired: 1 in, 3 out]
              n116 = Greater Or Equal To 0?(x=w288) -> (x >= 0?=w287:bool)
            }
            n117 = Index Array(array=w256, index=w259) -> (element=w255:path)
            n118 = call <vilib>:"Get LV Class Default Value.vi"("error in (no error)"=w275, "class path"=w255) -> ("error out"=w274:errorcluster, "object"=w278:refnum<class>)  [unwired: 8 in]
            n119 = To More Specific Class(target class=refnum<class "_Thermal Process Controller.lvclass"> refnum ("_Thermal Process Controller.lvclass"), reference=w278, error in=w274) -> (specific class reference=w277:refnum<class "_Thermal Process Controller.lvclass">, error out=w273:errorcluster)
            n120 = call-dynamic "Initialize--Method.vi"("error in (no error)"=w273, "VISA Resource"=w271, "_Thermal Process Controller in"=w277) -> ("error out"=w272:errorcluster, "Connected?"=w267:bool, "_Thermal Process Controller out"=w268:refnum<class "_Thermal Process Controller.lvclass">)  [unwired: 6 in]
            n121 = local read "Module ID"() -> (w264:i32)
            n122 = Bundle By Name(cluster=T19 {"Module ID"=0, "Ready"=FALSE, "error"={"status"=FALSE, "code"=0, "source"=""}} ("Start Up Process Controller (Reply Payload)"), "Module ID"=w264, "Ready"=w267) -> (w265:T19)
            n123 = Bundle By Name(cluster=w269, "_Thermal Process Controller"=w268) -> (w270:T2)
            n124 = case shown="True" w280 {
              tunnel: w281 -> [_ w293]
              tunnel: w265 -> [_ w292]
              tunnel: [_ w291] -> w279
              frame False {
              }
              frame True {
                n125 = Send Notification(notification=w292, notifier=w293) -> (error out=w291:errorcluster)  [unwired: 1 in, 1 out]
              }
            }
            n126 = call "Ready.vi"("error in"=w279, "Reply Payload"=w265) -> ()  [unwired: 9 in, 1 out]
          }
          frame "Shutdown Thermal Chamber" {
            # "Command the process controller to get to safe state to disconnect and then disconnect from process controller"
            n127 = Variant To Data(error in=w309, type=T7 {"Module ID"=-1, "Wait Notifier"=refnum, "wait for reply"=FALSE} ("Process Controller Shut Down Argument"), Variant=w308) -> (data=w306:T7, error out=w299:errorcluster)
            n128 = Unbundle By Name(w297) -> ("_Thermal Process Controller"=w300:refnum<class "_Thermal Process Controller.lvclass">)
            n129 = Unbundle By Name(w306) -> ("Wait Notifier"=w305:refnum<notifier>, "wait for reply"=w304:bool)
            n130 = call-dynamic "Shutdown--Method.vi"("error in (no error)"=w299, "_Thermal Process Controller in"=w300) -> ("error out"=w295:errorcluster, "Success?"=w294:bool, "_Thermal Process Controller out"=w296:refnum<class "_Thermal Process Controller.lvclass">)  [unwired: 7 in]
            n131 = local read "Module ID"() -> (w302:i32)
            n132 = Bundle By Name(cluster=T20 {"Module ID"=0, "Shutdown?"=FALSE, "error"={"status"=FALSE, "code"=0, "source"=""}} ("Process Controller Shut Down (Reply Payload)"), "Module ID"=w302, "Shutdown?"=w294) -> (w303:T20)
            n133 = Bundle By Name(cluster=w297, "_Thermal Process Controller"=w296) -> (w298:T2)
            n134 = case shown="True" w304 {
              tunnel: w305 -> [_ w312]
              tunnel: [_ w311] -> _
              tunnel: w303 -> [_ w310]
              frame False {
              }
              frame True {
                n135 = Send Notification(notification=w310, notifier=w312) -> (error out=w311:errorcluster)  [unwired: 1 in, 1 out]
              }
            }
          }
          frame "Set Temp Setpoint" {
            n136 = property class="Mod Admin"(reference=w313) -> ("Accessors:Module ID"=w314:i32)  [unwired: 1 in, 2 out]
            n137 = Unbundle By Name(w324) -> ("_Thermal Process Controller"=w323:refnum<class "_Thermal Process Controller.lvclass">)
            n138 = Variant To Data(error in=w334, type=T8 {"Module ID"=-1, "Temp Setpoint Data"={"Temp"=0.0, "Temp Units"=enum."Degrees F"}, "Wait Notifier"=refnum, "wait for reply"=FALSE} ("Set Temp Setpoint Argument"), Variant=w333) -> (data=w331:T8, error out=w326:errorcluster)
            n139 = Unbundle By Name(w331) -> ("Temp Setpoint Data"=w319:T9, "Wait Notifier"=w330:refnum<notifier>, "wait for reply"=w329:bool)
            n140 = call-dynamic "Set Temp Setpoint--Method.vi"("error in (no error)"=w326, "Temp Setpoint Data"=w319, "_Thermal Process Controller in"=w323) -> ("error out"=w322:errorcluster, "_Thermal Process Controller out"=w321:refnum<class "_Thermal Process Controller.lvclass">)  [unwired: 7 in]
            n141 = call-dynamic "Get Temp Setpoint--Method.vi"("error in (no error)"=w322, "Temp Setpoint Data"=w319, "_Thermal Process Controller in"=w321) -> ("error out"=w315:errorcluster, "Target Temp Setpoint"=w318:dbl, "_Thermal Process Controller out"=w320:refnum<class "_Thermal Process Controller.lvclass">)  [unwired: 5 in, 1 out]
            n142 = Bundle By Name(cluster=w319, "Temp"=w318) -> (w317:T9)
            n143 = Not(x=w315) -> (.not. x?=w316:bool)
            n144 = Bundle By Name(cluster=T21 {"Set?"=FALSE, "Temp Setpoint Data"={"Temp"=0.0, "Temp Units"=enum."Degrees F"}, "error"={"status"=FALSE, "code"=0, "source"=""}, "Module ID"=0} ("Set Temp Setpoint (Reply Payload)"), "Set?"=w316, "Temp Setpoint Data"=w317, "Module ID"=w314) -> (w328:T21)
            n145 = Bundle By Name(cluster=w324, "_Thermal Process Controller"=w320) -> (w325:T2)
            n146 = case shown="True" w329 {
              tunnel: w330 -> [_ w336]
              tunnel: w328 -> [_ w335]
              frame False {
              }
              frame True {
                n147 = Send Notification(notification=w335, notifier=w336) -> ()  [unwired: 1 in, 2 out]
              }
            }
          }
          frame "Set Temp Ramp Rate" {
            n148 = property class="Mod Admin"(reference=w337) -> ("Accessors:Module ID"=w338:i32)  [unwired: 1 in, 2 out]
            n149 = Unbundle By Name(w349) -> ("_Thermal Process Controller"=w346:refnum<class "_Thermal Process Controller.lvclass">)
            n150 = Variant To Data(error in=w358, type=T11 {"Module ID"=-1, "Temp Ramp Data"={"Temp Ramp Rate"=0.0, "Temp Units"=enum."Degrees F", "Rate Units"=enum."Degrees/Minutes"}, "Wait Notifier"=refnum, "wait for reply"=FALSE} ("Set Temp Ramp Rate Argument"), Variant=w357) -> (data=w355:T11, error out=w348:errorcluster)
            n151 = Unbundle By Name(w355) -> ("Temp Ramp Data"=w343:T12, "Wait Notifier"=w354:refnum<notifier>, "wait for reply"=w353:bool)
            n152 = call-dynamic "Set Temp Ramp Rate--Method.vi"("error in (no error)"=w348, "Temp Ramp Data"=w343, "_Thermal Process Controller in"=w346) -> ("error out"=w347:errorcluster, "_Thermal Process Controller out"=w345:refnum<class "_Thermal Process Controller.lvclass">)  [unwired: 7 in]
            n153 = call-dynamic "Get Temp Ramp Rate--Method.vi"("error in (no error)"=w347, "Temp Ramp Data"=w343, "_Thermal Process Controller in"=w345) -> ("error out"=w339:errorcluster, "Temp Ramp Rate"=w342:dbl, "_Thermal Process Controller out"=w344:refnum<class "_Thermal Process Controller.lvclass">)  [unwired: 6 in]
            n154 = Bundle By Name(cluster=w343, "Temp Ramp Rate"=w342) -> (w341:T12)
            n155 = Not(x=w339) -> (.not. x?=w340:bool)
            n156 = Bundle By Name(cluster=T22 {"Set?"=FALSE, "Temp Ramp Data"={"Temp Ramp Rate"=0.0, "Temp Units"=enum."Degrees F", "Rate Units"=enum."Degrees/Minutes"}, "error"={"status"=FALSE, "code"=0, "source"=""}, "Module ID"=0} ("Set Temp Ramp Rate (Reply Payload)"), "Set?"=w340, "Temp Ramp Data"=w341, "Module ID"=w338) -> (w352:T22)
            n157 = Bundle By Name(cluster=w349, "_Thermal Process Controller"=w344) -> (w350:T2)
            n158 = case shown="True" w353 {
              tunnel: w354 -> [_ w360]
              tunnel: w352 -> [_ w359]
              frame False {
              }
              frame True {
                n159 = Send Notification(notification=w359, notifier=w360) -> ()  [unwired: 1 in, 2 out]
              }
            }
          }
          frame "Set Temp Control State" {
            n160 = property class="Mod Admin"(reference=w361) -> ("Accessors:Module ID"=w362:i32)  [unwired: 1 in, 2 out]
            n161 = Variant To Data(error in=w381, type=T14 {"Module ID"=-1, "State"=FALSE, "Wait Notifier"=refnum, "wait for reply"=FALSE} ("Set Temp Control State Argument"), Variant=w380) -> (data=w378:T14, error out=w373:errorcluster)
            n162 = Unbundle By Name(w369) -> ("_Thermal Process Controller"=w368:refnum<class "_Thermal Process Controller.lvclass">)
            n163 = Unbundle By Name(w378) -> ("State"=w366:bool, "Wait Notifier"=w377:refnum<notifier>, "wait for reply"=w376:bool)
            n164 = call-dynamic "Set Temp Control--Method.vi"("error in (no error)"=w373, "Temp Control"=w366, "_Thermal Process Controller in"=w368) -> ("error out"=w372:errorcluster, "_Thermal Process Controller out"=w371:refnum<class "_Thermal Process Controller.lvclass">)  [unwired: 7 in]
            n165 = call-dynamic "Get Temp Control--Method.vi"("error in (no error)"=w372, "_Thermal Process Controller in"=w371) -> ("error out"=w364:errorcluster, "Temp Control"=w365:bool, "_Thermal Process Controller out"=w367:refnum<class "_Thermal Process Controller.lvclass">)  [unwired: 6 in, 1 out]
            n166 = Bundle By Name(cluster=w369, "_Thermal Process Controller"=w367) -> (w370:T2)
            n167 = Not(x=w364) -> (.not. x?=w363:bool)
            n168 = Bundle By Name(cluster=T23 {"Set?"=FALSE, "State"=FALSE, "error"={"status"=FALSE, "code"=0, "source"=""}, "Module ID"=0} ("Set Temp Control State (Reply Payload)"), "Set?"=w363, "State"=w365, "Module ID"=w362) -> (w375:T23)
            n169 = case shown="True" w376 {
              tunnel: w377 -> [_ w383]
              tunnel: w375 -> [_ w382]
              frame False {
              }
              frame True {
                n170 = Send Notification(notification=w382, notifier=w383) -> ()  [unwired: 1 in, 2 out]
              }
            }
          }
          frame "Get Temp Feedback" {
            n171 = property class="Mod Admin"(reference=w384) -> ("Accessors:Module ID"=w385:i32)  [unwired: 1 in, 2 out]
            n172 = Unbundle By Name(w394) -> ("_Thermal Process Controller"=w392:refnum<class "_Thermal Process Controller.lvclass">)
            n173 = Variant To Data(error in=w403, type=T15 {"Module ID"=-1, "Temp Units"=enum."Degrees F", "Wait Notifier"=refnum, "wait for reply"=FALSE} ("Get Temp Feedback Argument"), Variant=w402) -> (data=w400:T15, error out=w395:errorcluster)
            n174 = Unbundle By Name(w400) -> ("Temp Units"=w388:T10, "Wait Notifier"=w399:refnum<notifier>, "wait for reply"=w398:bool)
            n175 = call-dynamic "Get Temp Feedback--Method.vi"("error in (no error)"=w395, "Temp Units"=w388, "_Thermal Process Controller in"=w392) -> ("error out"=w387:errorcluster, "Temp Feedback"=w389:dbl, "_Thermal Process Controller out"=w391:refnum<class "_Thermal Process Controller.lvclass">)  [unwired: 6 in]
            n176 = Bundle By Name(cluster=T9 {"Temp"=0.0, "Temp Units"=enum."Degrees F"} ("Temp Feedback Data"), "Temp"=w389, "Temp Units"=w388) -> (w386:T9)
            n177 = Bundle By Name(cluster=T24 {"Temp Feedback Data"={"Temp"=0.0, "Temp Units"=enum."Degrees F"}, "error"={"status"=FALSE, "code"=0, "source"=""}, "Module ID"=0} ("Get Temp Feedback (Reply Payload)"), "Temp Feedback Data"=w386, "Module ID"=w385) -> (w397:T24)
            n178 = Bundle By Name(cluster=w394, "_Thermal Process Controller"=w391) -> (w393:T2)
            n179 = case shown="True" w398 {
              tunnel: w399 -> [_ w405]
              tunnel: w397 -> [_ w404]
              frame False {
              }
              frame True {
                n180 = Send Notification(notification=w404, notifier=w405) -> ()  [unwired: 1 in, 2 out]
              }
            }
          }
          frame "Read Controller Data" {
            w412 = T9 {"Temp"=0.0, "Temp Units"=enum."Degrees F"} ("Chamber Temp")
            n181 = property class="Mod Admin"(reference=w406) -> ("Accessors:Module ID"=w407:i32)  [unwired: 1 in, 2 out]
            n182 = Unbundle By Name(w425) -> ("_Thermal Process Controller"=w417:refnum<class "_Thermal Process Controller.lvclass">)
            n183 = Variant To Data(error in=w434, type=T16 {"Module ID"=-1, "Temp Units"=enum."Degrees F", "Wait Notifier"=refnum, "wait for reply"=FALSE} ("Read Controller Data Argument"), Variant=w433) -> (data=w431:T16, error out=w422:errorcluster)
            n184 = Unbundle By Name(w431) -> ("Temp Units"=w414:T10, "Wait Notifier"=w430:refnum<notifier>, "wait for reply"=w429:bool)
            n185 = call-dynamic "Get Temp Feedback--Method.vi"("error in (no error)"=w422, "Temp Units"=w414, "_Thermal Process Controller in"=w417) -> ("error out"=w421:errorcluster, "Temp Feedback"=w418:dbl, "_Thermal Process Controller out"=w416:refnum<class "_Thermal Process Controller.lvclass">)  [unwired: 6 in]
            n186 = Bundle By Name(cluster=T9 {"Temp"=0.0, "Temp Units"=enum."Degrees F"} ("Temp Setpoint Data"), "Temp Units"=w414) -> (w423:T9)
            n187 = Bundle(cluster=w412, "Temp"=w418, "Temp Units"=w414) -> (w410:T9)
            n188 = call-dynamic "Get Temp Setpoint--Method.vi"("error in (no error)"=w421, "Temp Setpoint Data"=w423, "_Thermal Process Controller in"=w416) -> ("error out"=w420:errorcluster, "Actual Temp Setpoint"=w413:dbl, "_Thermal Process Controller out"=w419:refnum<class "_Thermal Process Controller.lvclass">)  [unwired: 5 in, 1 out]
            n189 = Bundle(cluster=w412, "Temp"=w413, "Temp Units"=w414) -> (w411:T9)
            n190 = call-dynamic "Get Temp Control--Method.vi"("error in (no error)"=w420, "_Thermal Process Controller in"=w419) -> ("error out"=w408:errorcluster, "Output"=w415:dbl, "_Thermal Process Controller out"=w409:refnum<class "_Thermal Process Controller.lvclass">)  [unwired: 6 in, 1 out]
            n191 = Bundle By Name(cluster=T25 {"Chamber Temp"={"Temp"=0.0, "Temp Units"=enum."Degrees F"}, "Temp Setpoint"={"Temp"=0.0, "Temp Units"=enum."Degrees F"}, "Chamber Output"=0.0, "error"={"status"=FALSE, "code"=0, "source"=""}, "Module ID"=0} ("Read Controller Data (Reply Payload)"), "Chamber Temp"=w410, "Temp Setpoint"=w411, "Chamber Output"=w415, "Module ID"=w407) -> (w428:T25)
            n192 = Bundle By Name(cluster=w425, "_Thermal Process Controller"=w409) -> (w426:T2)
            n193 = case shown="True" w429 {
              tunnel: w430 -> [_ w436]
              tunnel: w428 -> [_ w435]
              frame False {
              }
              frame True {
                n194 = Send Notification(notification=w435, notifier=w436) -> ()  [unwired: 1 in, 2 out]
              }
            }
          }
          frame "---Copy This Frame---" {
            # "Duplicate this frame when creating new messages.  Change this comment in the duplicated frame to describe this message."
            n195 = Merge Errors(w439) -> (w438:errorcluster)
          }
          frame "---Exit and Error Handling---" {
            # "Separator - the following cases handle errors and exit messages."
          }
          frame "Error" {
            # "#CodeRecommended - If you ever change the name of this \"Error\" message, you'll need to update the name in the Check Loop Error.vi as well."
            # "#CodeRecommended - If the module is running in standalone mode (External Launch = FALSE), this code will pop up an error dialog and call the 'Exit' message if an error occurs. Add more fine-grained error handling here."
            # "Error - Check the error message data and respond accordingly. This message is sent by the \"Error Handler\" VIs at the end of each loop in this application."
            n196 = property on="Property Node" class="Mod Admin"(reference=w445) -> ("Accessors:External Launch"=w444:bool, "Accessors:Module ID"=w442:i32)  [unwired: 1 in, 2 out]
            n197 = Variant To Data(error in=w452, type=errorcluster {"status"=FALSE, "code"=0, "source"=""} ("error constant"), Variant=w446) -> (data=w453:errorcluster, error out=w450:errorcluster)
            n198 = call "Error Reported.vi"("Error"=w453, "Module ID"=w442) -> ()  [unwired: 9 in, 1 out]
            n199 = case shown="True" w444 {
              tunnel: [w458 _] -> w449
              tunnel: w443 -> [w456 _]
              tunnel: w453 -> [w457 _]
              frame False {
                # "If the module is running standalone, then pop up an error dialog and call the \"Exit\" message."
                n200 = call <vilib>:"Simple Error Handler.vi"("error in (no error)"=w457) -> ()  [unwired: 4 in, 5 out]
                n201 = call-poly <vilib>:"Delacor_lib_QMH_Enqueue Message (poly).vi"("Priority Message? (F)"=TRUE, "Message"="Exit", "Message Queue in"=w456) -> ("error out"=w458:errorcluster)  [unwired: 7 in, 1 out]
              }
              frame True {
                # "If the module was launched externally, calling the Error Reported broadcast VI is the only action performed by the \"Error\" message. The module's caller can then process the error appropriately."
              }
            }
            n202 = Merge Errors(w450, w449) -> (w448:errorcluster)
            n203 = local write "error out"(w448) -> ()
          }
          frame "Simulate MHL Error" {
            # "#DQMH_HowTo The 'Simulate MHL Error' button  illustrates how the MHL handles errors. This event is instructional in nature and can be removed."
            # "Simulate an error occurring at the MHL"
            n204 = property on="Property Node" class="Mod Admin"(reference=w460) -> ("Accessors:Module ID"=w461:i32)  [unwired: 1 in, 2 out]
            n205 = call "Module Name--constant.vi"("Module ID"=w461) -> ("Module Name"=w459:string)  [unwired: 10 in]
            n206 = xnode "Error Ring"("parameter 0"=w459) -> ("error out"=w463:errorcluster)
            n207 = Merge Errors(w465, w463) -> (w464:errorcluster)
          }
          frame "Exit" {
            w480 = 91  # 91: not all Exit messages will have an argument
            w481 = TRUE  # Stop the VI
            # "Release the message queue reference"
            # "#CodeNeeded - Add any required cleanup code here."
            # "Exit - Exit the application."
            n208 = Variant To Data(error in=w489, type=T4 {"Module ID"=-1, "Origin"="", "Exit via Stop Module Req?"=FALSE, "Wait for Module to stop?"=FALSE} ("Stop Argument"), Variant=w479) -> (data=w476:T4, error out=w484:errorcluster)
            n209 = call <vilib>:"Clear Errors.vi"("error in (no error)"=w484, "specific error code to clear (0: all)"=w480) -> ("error out"=w488:errorcluster)  [unwired: 4 in, 1 out]
            n210 = control-ref of="This VI"() -> (w474:refnum<vi>)
            n211 = call-dynamic "Delacor_lib_QMH_Release Message Queue.vi"("error in"=w488, "Message Queue"=w483) -> ("error out"=w487:errorcluster)  [unwired: 9 in]
            n212 = call "Handle Exit.vi"("Stop Argument"=w476, "Module Admin in"=w475, "VI reference"=w474) -> ("error out"=w485:errorcluster, "Wait for Stop?"=w477:bool)  [unwired: 7 in]
            n213 = property class="Mod Admin"(reference=w475) -> ("Accessors:Module ID"=w473:i32)  [unwired: 1 in, 2 out]
            n214 = Merge Errors(w487, w485) -> (w486:errorcluster)
            n215 = call "Error Reported.vi"("Error"=w486, "Module ID"=w473) -> ()  [unwired: 9 in, 1 out]
          }
          frame Default {
            # "'Default' case only runs if there is a message that isn't defined in any of the other cases.  Output a programming error."
            n216 = property on="Property Node" class="Mod Admin"(reference=w491) -> ("Accessors:Module ID"=w490:i32)  [unwired: 1 in, 2 out]
            n217 = call "Module Name--constant.vi"("Module ID"=w490) -> ("Module Name"=w492:string)  [unwired: 10 in]
            n218 = xnode "Error Ring"("parameter 0"=w493, "parameter 1"=w492) -> ("error out"=w497:errorcluster)
            n219 = Merge Errors(w495, w497) -> (w496:errorcluster)
          }
        }
        n220 = call-dynamic "Delacor_lib_QMH_Error Handler - Message Handling Loop.vi"("error in"=w231, "Message Queue in"=w221) -> ("dup error in"=w228:errorcluster)  [unwired: 8 in, 1 out]
      }
    }
    frame Error {
      n221 = call "Synchronize Caller Events.vi"("Module Admin"=w511) -> ("Module Admin out"=w510:refnum<class "Delacor_lib_QMH_Cloneable Module Admin.lvclass">)  [unwired: 9 in, 1 out]
      n222 = property on="Property Node" class="Mod Admin"(reference=w510) -> ("Accessors:Module ID"=w509:i32)  [unwired: 1 in, 2 out]
      n223 = call-dynamic "Delacor_lib_QMH_Release Message Queue.vi"("error in"=w508, "Message Queue"=w506) -> ("error out"=w507:errorcluster)  [unwired: 9 in]
      n224 = call "Module Name--constant.vi"("Module ID"=w509) -> ("Module Name"=w514:string)  [unwired: 10 in]
      n225 = Format Into String(format string="An error occurred during initialization. %s is no longer running.", w514) -> (resulting string=w512:string)  [unwired: 2 in, 1 out]
      n226 = call "Error Reported.vi"("Additional Information"=w512, "Error"=w507, "Module ID"=w509) -> ()  [unwired: 8 in, 1 out]
    }
  }
  n227 = Merge Errors(w17, w16) -> (w18:errorcluster)
  n228 = call "Close Module.vi"("error in"=w18, "Wait for stop?"=w2, "Module Admin in"=w4) -> ("error out"=w14:errorcluster, "External Launch"=w1:bool, "Module Admin out"=w3:refnum<class "Delacor_lib_QMH_Cloneable Module Admin.lvclass">)  [unwired: 6 in]
  n229 = Unregister For Events(event registration refnum=w9, error in=w14) -> (error out=w13:errorcluster)
  "error out" <- w13
  n230 = case "External Launch?" shown="True" w1 {
    tunnel: w13 -> [_ w516]
    frame False {
    }
    frame True {
      n231 = case shown="No Error" w516 {
        frame No Error {
          n232 = invoke class="VI" method="FP.Close"() -> ()  [unwired: 3 in, 3 out]
        }
        frame Error {
          n233 = invoke class="VI" method="FP.Open"("Activate"=TRUE ("Activate?")) -> ()  [unwired: 4 in, 5 out]
        }
      }
    }
  }
  n234 = local write "Module Admin"(w3) -> ()
